vi "LDO Terminate Conditions.vi"(8 "error in (no error)":errorcluster, 10 "Event Booleans":T1, 11 "All Data":T2 {"PLC Data"."PLC Data - LDO"."Timing"."Absolute Time" format="%<%H:%M:%S%3u>t"; "PLC Data"."PLC Data - LDO"."Timing"."Display Time" format="%#.20f"; "PLC Data"."PLC Data - LDO"."Timing"."Test Time Ref" format="%#.20f"; "PLC Data"."PLC Data - LDO"."Timing"."Precondition Time Ref" format="%#.20f"; "PLC Data"."PLC Data - LDO"."Timing"."First Call Time Ref" format="%#.20f"; "PLC Data"."PLC Data - FVIR"."Timing"."Absolute Time" format="%<%H:%M:%S%3u>t"; "PLC Data"."PLC Data - FVIR"."Timing"."Display Time" format="%#.20f"; "PLC Data"."PLC Data - FVIR"."Timing"."Test Time Ref" format="%#.20f"; "PLC Data"."PLC Data - FVIR"."Timing"."Precondition Time Ref" format="%#.20f"; "PLC Data"."PLC Data - FVIR"."Timing"."First Call Time Ref" format="%#.20f"}) -> (0 "error out":errorcluster, 2 "Event Booleans Out":T1, 3 "All Data Out":T2 {"PLC Data"."PLC Data - LDO"."Timing"."Absolute Time" format="%<%H:%M:%S%3u>t"; "PLC Data"."PLC Data - LDO"."Timing"."Display Time" format="%#.20f"; "PLC Data"."PLC Data - LDO"."Timing"."Test Time Ref" format="%#.20f"; "PLC Data"."PLC Data - LDO"."Timing"."Precondition Time Ref" format="%#.20f"; "PLC Data"."PLC Data - LDO"."Timing"."First Call Time Ref" format="%#.20f"; "PLC Data"."PLC Data - FVIR"."Timing"."Absolute Time" format="%<%H:%M:%S%3u>t"; "PLC Data"."PLC Data - FVIR"."Timing"."Display Time" format="%#.20f"; "PLC Data"."PLC Data - FVIR"."Timing"."Test Time Ref" format="%#.20f"; "PLC Data"."PLC Data - FVIR"."Timing"."Precondition Time Ref" format="%#.20f"; "PLC Data"."PLC Data - FVIR"."Timing"."First Call Time Ref" format="%#.20f"})   [LabVIEW 2020]
uses:
  Modbus/Modbus All Data.ctl
  Modbus/Modbus PLC Data All.ctl
  Modbus/Modbus FVIR Control.ctl
  Modbus/Modbus Timing.ctl
  <vilib>/Utility/miscctls.llb/LVDateTimeRec.ctl
  Modbus/Modbus LDO Control.ctl
  WritingDataFile/Data to Save.ctl
  Terminate Conditions Cluster.ctl
  Drivers/Inficon Transmitter/Type Definitions/Inficon Data.ctl
  Modbus/Modbus Gas Meter Data.ctl
  Drivers/Alicat LabVIEW Drivers 2v1/Sub-VIs/Data Cluster.ctl
  Drivers/Alicat LabVIEW Drivers 2v1/Sub-VIs/Units of Measure.ctl
  Gas_Rate/HEWH ANSI Rate.ctl
  Drivers/Resideo Gas Valve/Type Definitions/Vesta Info.ctl
  Event Booleans.ctl
panel:
  # "Totalizer Timer"
  # "Totalizer Timer"
  # "Natural Gas"
  # "Propane"
  # "Totalizer Timer"
  # "Totalizer Timer"
  # "Natural Gas"
  # "Propane"
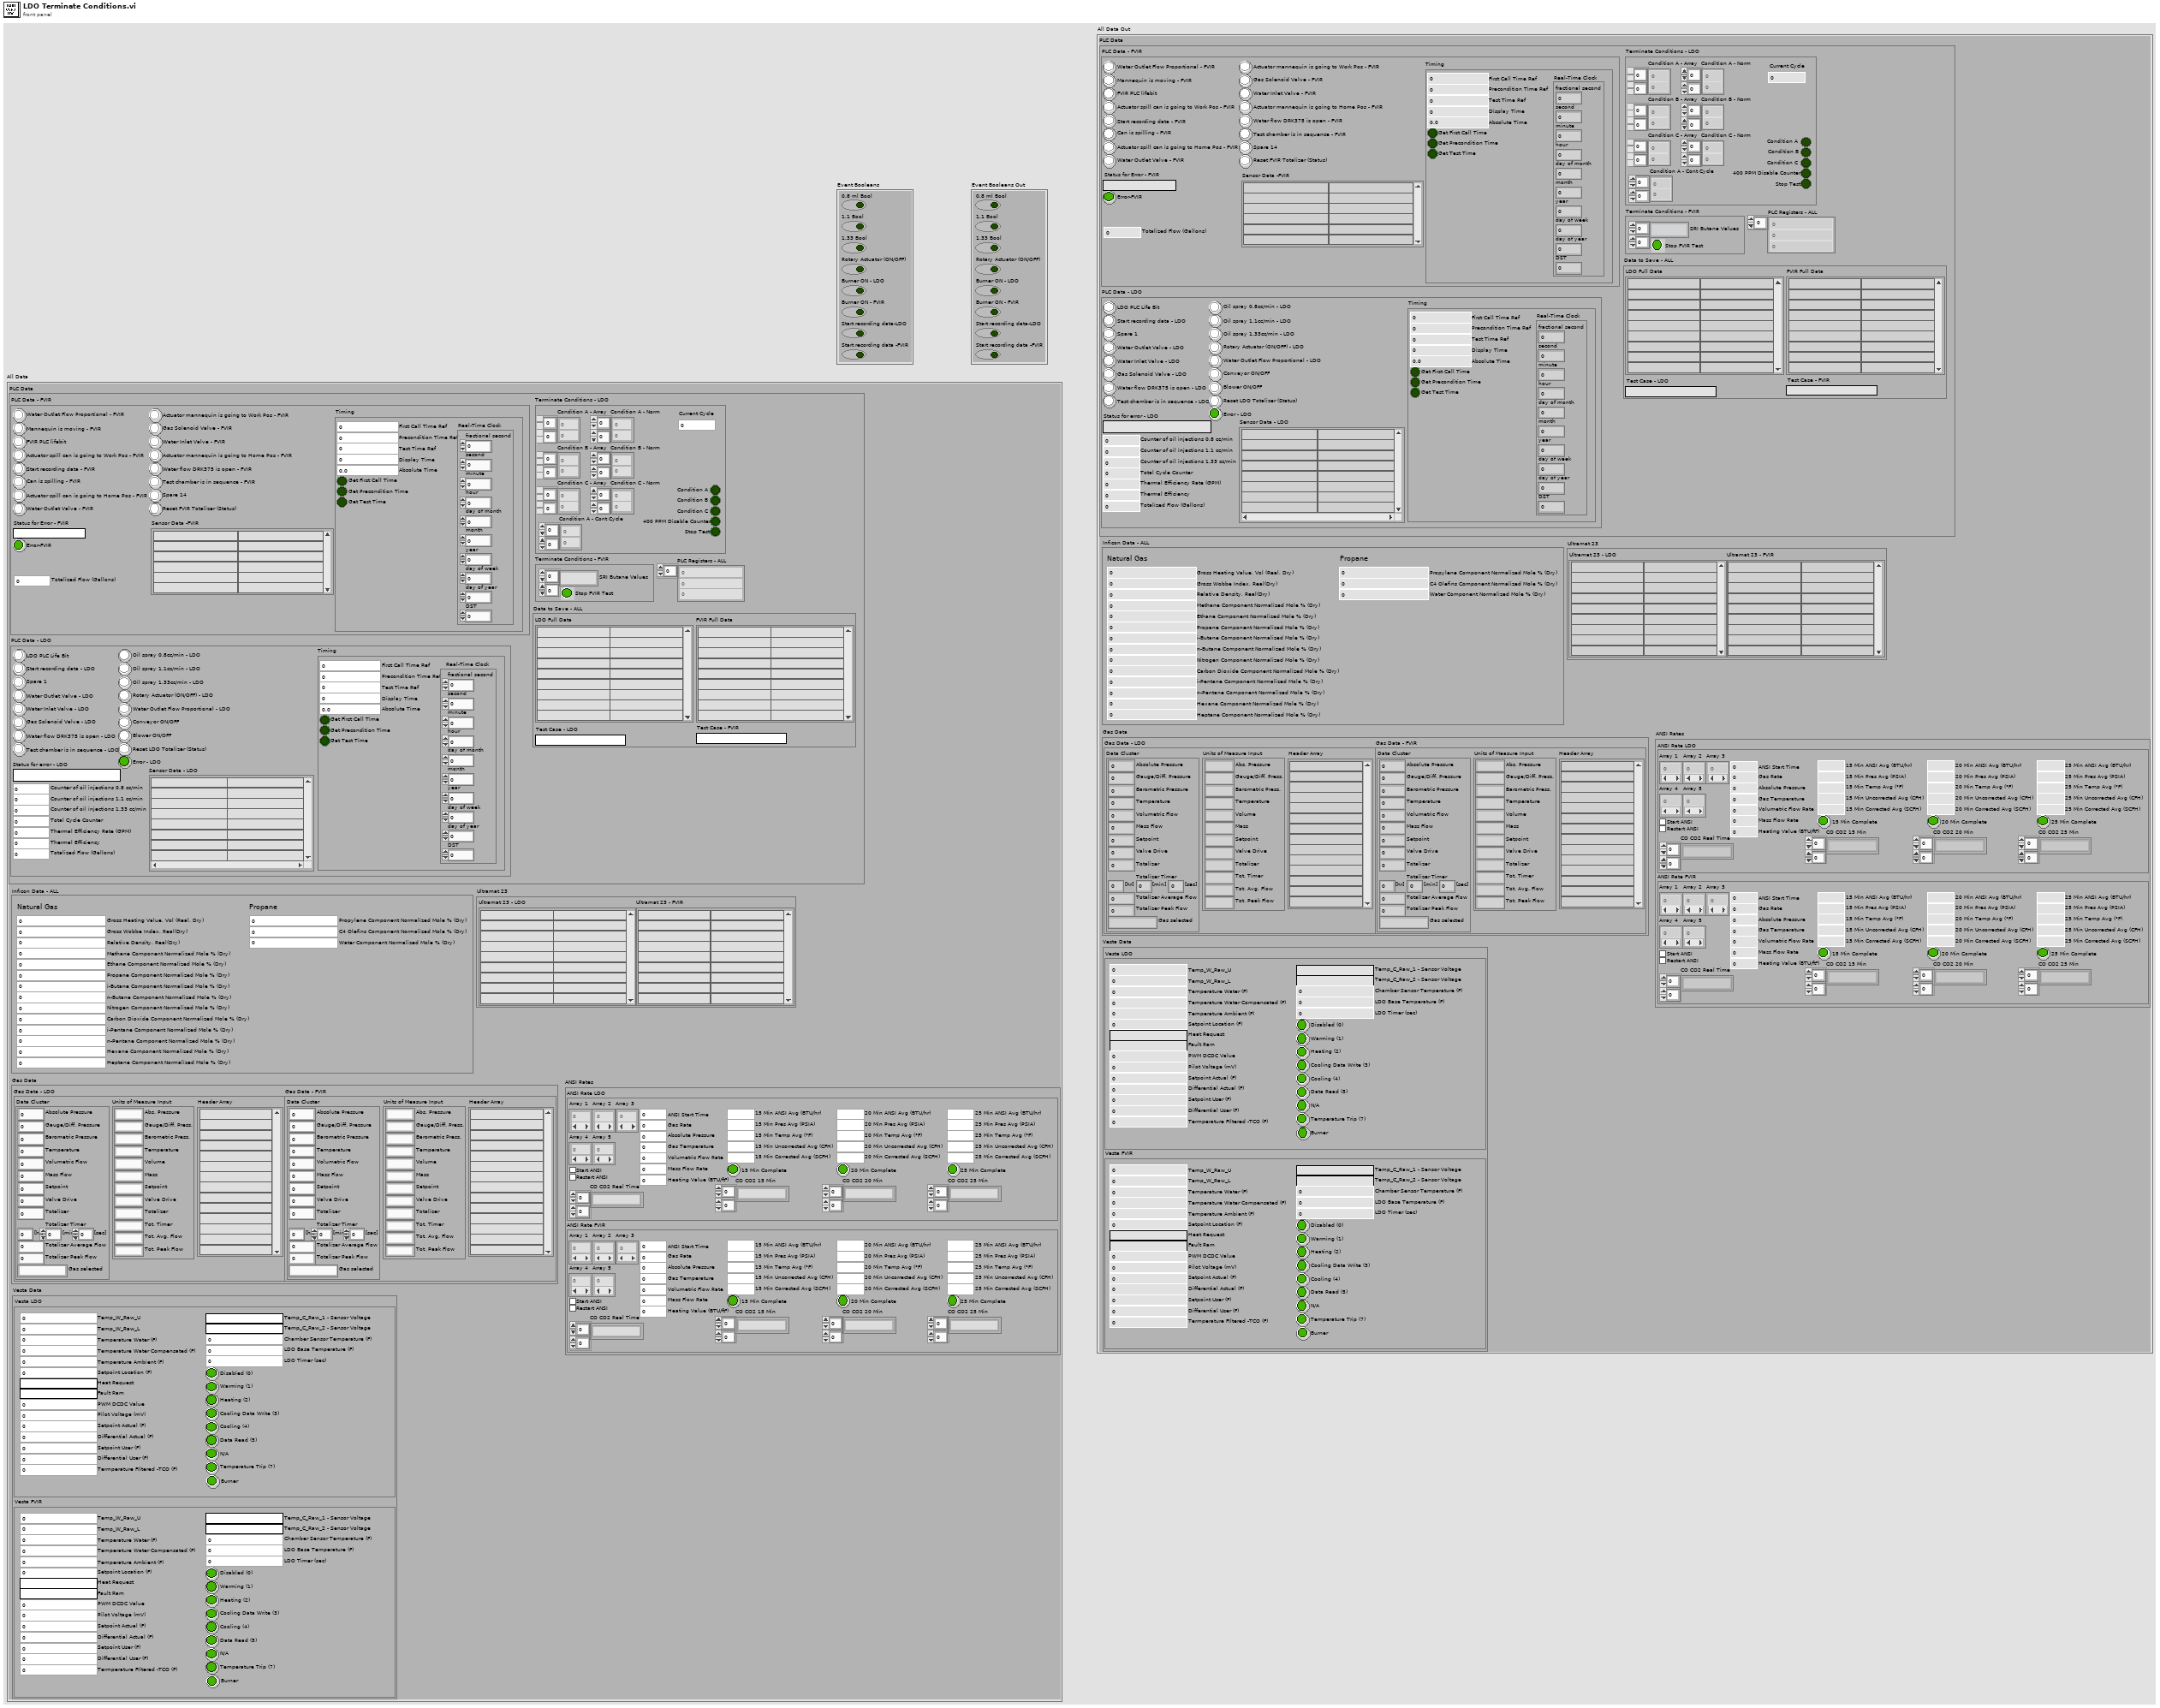
[diagram p1: front panel]
types:
  T1 = typedef "Event Booleans.ctl" = cluster{"Burner ON - LDO":bool, "0.8 ml Bool":bool, "1.1 Bool":bool, "1.33 Bool":bool, "Start recording data-LDO":bool, "Rotary Actuator (ON/OFF)":bool, "Burner ON - FVIR":bool, "Start recording data -FVIR ":bool}
  T2 = typedef "Modbus All Data.ctl" = cluster{"PLC Data":T3, "Inficon Data - ALL":T10, "Gas Data":cluster{"Gas Data - LDO":T11, "Gas Data - FVIR":T11}, "Ultramat 23":cluster{"Ultramat 23 - LDO":string[][], "Ultramat 23 - FVIR":string[][]}, "ANSI Rates":cluster{"ANSI Rate LDO":T14, "ANSI Rate FVIR":T14}, "Vesta Data":cluster{"Vesta LDO":T15, "Vesta FVIR":T15}}
  T3 = typedef "Modbus PLC Data All.ctl" = cluster{"PLC Data - FVIR":T4, "PLC Data - LDO":T7, "PLC Registers - ALL":i16[], "Data to Save - ALL":T8, "Terminate Conditions - LDO":T9, "Terminate Conditions - FVIR":cluster{"SRI Butane Values":string[][], "Stop FVIR Test":bool}}
  T4 = typedef "Modbus FVIR Control.ctl" = cluster{"Reset FVIR Totalizer (Status)":bool, "Spare 14":bool, "Actuator mannequin is going to Work Pos - FVIR":bool, "Actuator mannequin is going to Home Pos - FVIR":bool, "Test chamber is in sequence - FVIR ":bool, "Water flow DRK375 is open - FVIR":bool, "Gas Solenoid Valve - FVIR":bool, "Water Inlet Valve - FVIR":bool, "Water Outlet Flow Proportional - FVIR":bool, "Start recording data - FVIR":bool, "Actuator spill can is going to Work Pos - FVIR":bool, "Actuator spill can is going to Home Pos - FVIR":bool, "Water Outlet Valve - FVIR":bool, "Can is spilling - FVIR":bool, "Mannequin is moving - FVIR":bool, "FVIR PLC lifebit":bool, "Status for Error - FVIR":string, "Error-FVIR":bool, "Sensor Data -FVIR":string[][], "Totalized Flow (Gallons)":dbl, "Timing":T5}
  T5 = typedef "Modbus Timing.ctl" = cluster{"First Call Time Ref":dbl, "Precondition Time Ref":dbl, "Test Time Ref":dbl, "Get First Call Time":bool, "Get Precondition Time":bool, "Get Test Time":bool, "Display Time":dbl, "Real-Time Clock":T6, "Absolute Time":dbl}
  T6 = typedef "LVDateTimeRec.ctl" = cluster{"fractional second":dbl, "second":i32, "minute":i32, "hour":i32, "day of month":i32, "month":i32, "year":i32, "day of week":i32, "day of year":i32, "DST":i32}
  T7 = typedef "Modbus LDO Control.ctl" = cluster{"LDO PLC Life Bit":bool, "Start recording data - LDO":bool, "Spare 1":bool, "Water Outlet Valve - LDO":bool, "Water Inlet Valve - LDO":bool, "Gas Solenoid Valve - LDO":bool, "Water flow DRK375 is open - LDO":bool, "Test chamber is in sequence - LDO":bool, "Oil spray 0.8cc/min - LDO":bool, "Oil spray 1.1cc/min - LDO":bool, "Oil spray 1.33cc/min - LDO":bool, "Rotary Actuator (ON/OFF) - LDO":bool, "Water Outlet Flow Proportional - LDO":bool, "Conveyor ON/OFF":bool, "Blower ON/OFF":bool, "Reset LDO Totalizer (Status)":bool, "Status for error - LDO":string, "Error - LDO":bool, "Sensor Data - LDO":string[][], "Thermal Efficiency Rate (GPM)":dbl, "Thermal Efficiency":dbl, "Totalized Flow (Gallons)":dbl, "Counter of oil injections 1.33 cc/min":u16, "Total Cycle Counter":u16, "Counter of oil injections 1.1 cc/min":u16, "Counter of oil injections 0.8 cc/min":u16, "Timing":T5}
  T8 = typedef "Data to Save.ctl" = cluster{"LDO Full Data":string[][], "FVIR Full Data":string[][], "Test Case - FVIR":string, "Test Case - LDO":string}
  T9 = typedef "Terminate Conditions Cluster.ctl" = cluster{"Condition B - Array":dbl[][], "Current Cycle":u16, "Condition C - Array":dbl[][], "Condition A - Array":dbl[][], "400 PPM Disable Counter":bool, "Condition A - Norm":dbl[][], "Condition B - Norm":dbl[][], "Condition C - Norm":dbl[][], "Condition A":bool, "Condition B":bool, "Condition C":bool, "Condition A - Cont Cycle":dbl[][], "Stop Test":bool}
  T10 = typedef "Inficon Data.ctl" = cluster{"Gross Heating Value, Vol (Real, Dry)":dbl, "Nitrogen Component Normalized Mole % (Dry)":dbl, "Methane Component Normalized Mole % (Dry)":dbl, "Carbon Dioxide Component Normalized Mole % (Dry)":dbl, "Ethane Component Normalized Mole % (Dry)":dbl, "Propane Component Normalized Mole % (Dry)":dbl, "i-Pentane Component Normalized Mole % (Dry)":dbl, "i-Butane Component Normalized Mole % (Dry)":dbl, "n-Butane Component Normalized Mole % (Dry)":dbl, "n-Pentane Component Normalized Mole % (Dry)":dbl, "Hexane Component Normalized Mole % (Dry)":dbl, "Heptane Component Normalized Mole % (Dry)":dbl, "Gross Wobbe Index, Real(Dry)":dbl, "Relative Density, Real(Dry)":dbl, "Propylene Component Normalized Mole % (Dry)":dbl, "C4 Olefins Component Normalized Mole % (Dry)":dbl, "Water Component Normalized Mole % (Dry)":dbl}
  T11 = typedef "Modbus Gas Meter Data.ctl" = cluster{"Data Cluster":T12, "Units of Measure Input":T13, "Header Array":string[]}
  T12 = typedef "Data Cluster.ctl" = cluster{"Absolute Pressure":dbl, "Gauge/Diff. Pressure":dbl, "Barometric Pressure":dbl, "Temperature":dbl, "Volumetric Flow":dbl, "Mass Flow":dbl, "Setpoint":dbl, "Valve Drive":dbl, "Totalizer":dbl, "[hr]":dbl, "[min]":dbl, "[sec]":dbl, "Totalizer Average Flow":dbl, "Totalizer Peak Flow":dbl, "Gas selected":string}
  T13 = typedef "Units of Measure.ctl" = cluster{"Abs. Pressure":string, "Gauge/Diff. Press.":string, "Barometric Press.":string, "Temperature":string, "Volume":string, "Mass":string, "Setpoint":string, "Valve Drive":string, "Totalizer":string, "Tot. Timer":string, "Tot. Avg. Flow":string, "Tot. Peak Flow":string}
  T14 = typedef "HEWH ANSI Rate.ctl" = cluster{"Array 1":dbl[], "Array 3":dbl[], "Array 2":dbl[], "Start ANSI":bool, "ANSI Start Time":dbl, "Restart ANSI":bool, "15 Min ANSI Avg (BTU/hr)":dbl, "20 Min ANSI Avg (BTU/hr)":dbl, "25 Min ANSI Avg (BTU/hr)":dbl, "Absolute Pressure":dbl, "Gas Temperature":dbl, "Volumetric Flow Rate":dbl, "Mass Flow Rate":dbl, "Array 4":dbl[], "Array 5":dbl[], "Gas Rate":dbl, "15 Min Pres Avg (PSIA)":dbl, "20 Min Pres Avg (PSIA)":dbl, "25 Min Pres Avg (PSIA)":dbl, "15 Min Temp Avg (°F) ":dbl, "20 Min Temp Avg (°F)":dbl, "25 Min Temp Avg (°F)":dbl, "15 Min Uncorrected Avg (CFH)":dbl, "20 Min Uncorrected Avg (CFH)":dbl, "25 Min Uncorrected Avg (CFH)":dbl, "15 Min Corrected Avg (SCFH)":dbl, "20 Min Corrected Avg (SCFH)":dbl, "25 Min Corrected Avg (SCFH)":dbl, "15 Min Complete":bool, "20 Min Complete":bool, "25 Min Complete":bool, "Heating Value (BTU/ft³)":dbl, "CO CO2 15 Min":string[][], "CO CO2 20 Min":string[][], "CO CO2 25 Min":string[][], "CO CO2 Real Time":string[][]}
  T15 = typedef "Vesta Info.ctl" = cluster{"Temp_W_Raw_U":u16, "Temp_W_Raw_L":u16, "Temperature Water (F)":dbl, "Temperature Water Compensated (F)":dbl, "Temperature Ambient (F)":dbl, "Setpoint Location (F)":dbl, "Heat Request":string, "Fault Ram":string, "PWM DCDC Value":u16, "Pilot Voltage (mV)":dbl, "Setpoint Actual (F)":dbl, "Differential Actual (F)":dbl, "Setpoint User (F)":dbl, "Differential User (F)":dbl, "Termperature FIltered -TCO (F)":dbl, "Temp_C_Raw_1 - Sensor Voltage":string, "Temp_C_Raw_2 - Sensor Voltage":string, "Chamber Sensor Temperature (F)":dbl, "LDO Base Temperature (F)":dbl, "LDO Timer (sec)":i16, "Disabled (0)":bool, "Warming (1)":bool, "Heating (2)":bool, "Cooling Data Write (3)":bool, "Cooling (4)":bool, "Data Read (5)":bool, "N/A":bool, "Temperature Trip (7)":bool, "Burner":bool}
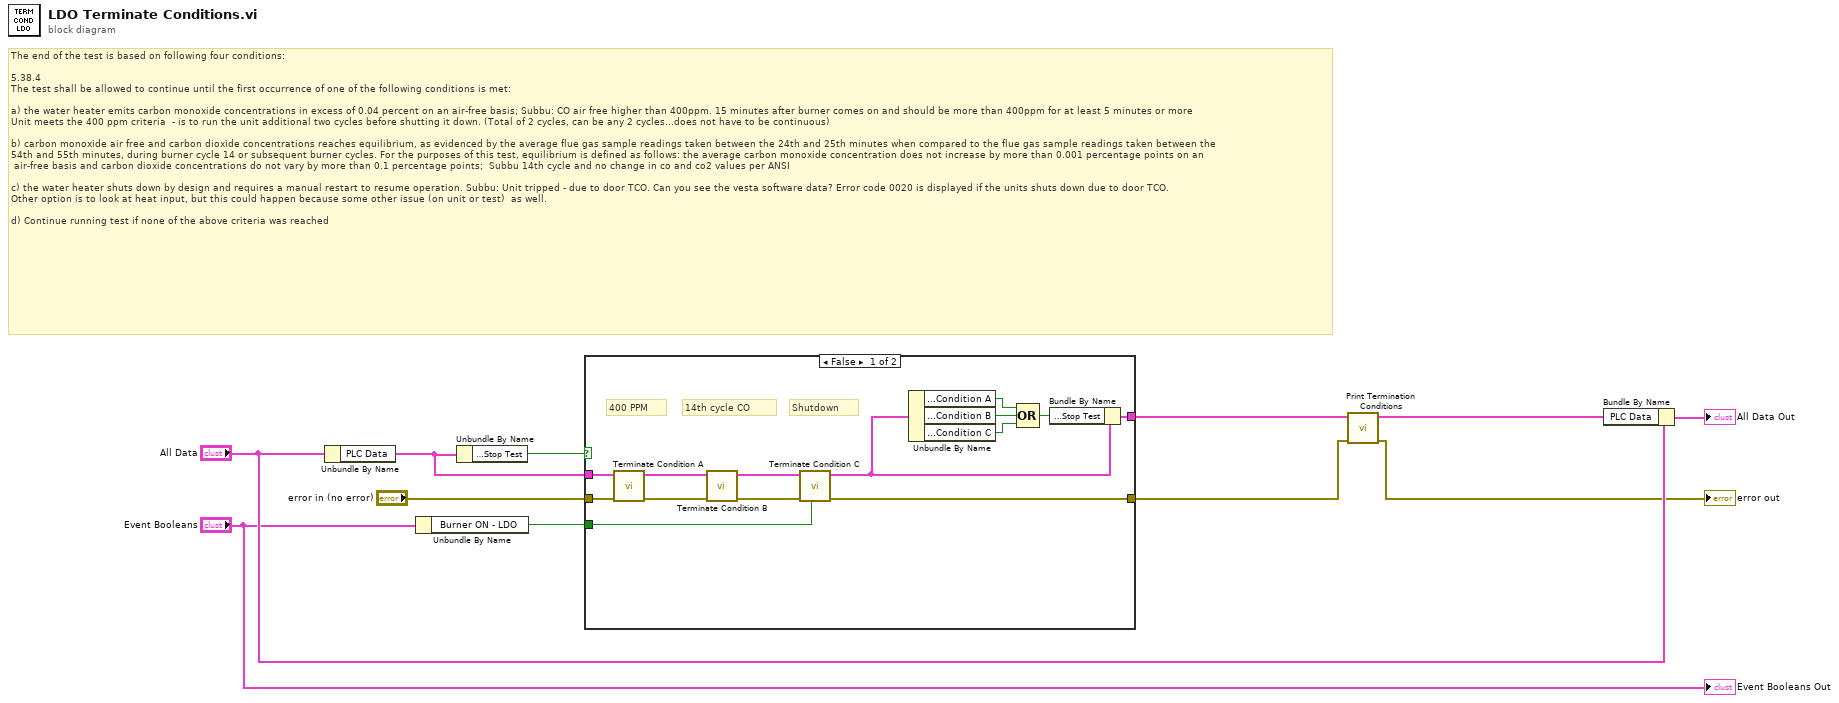
[diagram p0: block diagram]
diagram:
  # "The end of the test is based on following four conditions:\n\n5.38.4\nThe test shall be allowed to continue until the first occurrence of one of the following conditions is met: \n\na) the water heater emits carbon monoxide concentrations in excess of 0.04 percent on an air-free basis; Subbu: CO air free higher than 400ppm. 15 minutes after burner comes on and should be more than 400ppm for at least 5 minutes or more\nUnit meets the 400 ppm criteria  - is to run the unit additional two cycles before shutting it down. (Total of 2 cycles, can be any 2 cycles...does not have to be continuous)\n\nb) carbon monoxide air free and carbon dioxide concentrations reaches equilibrium, as evidenced by the average flue gas sample readings taken between the 24th and 25th minutes when compared to the flue gas sample readings taken between the\n54th and 55th minutes, during burner cycle 14 or subsequent burner cycles. For the purposes of this test, equilibrium is defined as follows: the average carbon monoxide concentration does not increase by more than 0.001 percentage points on an\n air-free basis and carbon dioxide concentrations do not vary by more than 0.1 percentage points;  Subbu 14th cycle and no change in co and co2 values per ANSI\n\nc) the water heater shuts down by design and requires a manual restart to resume operation. Subbu: Unit tripped - due to door TCO. Can you see the vesta software data? Error code 0020 is displayed if the units shuts down due to door TCO. \nOther option is to look at heat input, but this could happen because some other issue (on unit or test)  as well.\n\nd) Continue running test if none of the above criteria was reached"
  n1 = Unbundle By Name("All Data") -> ("PLC Data"=w9:T3)
  n2 = Unbundle By Name("Event Booleans") -> ("Burner ON - LDO"=w6:bool)
  n3 = Unbundle By Name(w9) -> ("Terminate Conditions - LDO.Stop Test"=w10:bool)
  n4 = case shown="False" w10 {
    tunnel: w6 -> [w25 _]
    tunnel: w9 -> [w24 w27]
    tunnel: [w21 w26] -> w2
    tunnel: "error in (no error)" -> [w20 w26]
    tunnel: [w13 w27] -> w4
    frame False {
      # "Shutdown"
      # "14th cycle CO"
      # "400 PPM"
      n5 = call "Terminate Condition A.vi"("error in"=w20, "PLC Data In"=w24) -> ("error out"=w23:errorcluster, "PLC Data Out"=w19:T3)  [unwired: 8 in]
      n6 = call "Terminate Condition B.vi"("error in (no error)"=w23, "PLC Data Out in"=w19) -> ("error out"=w22:errorcluster, "PLC Data Out out"=w18:T3)  [unwired: 8 in]
      n7 = call "Terminate Condition C.vi"("Burner ON"=w25, "error in"=w22, "PLC Data In"=w18) -> ("error out"=w21:errorcluster, "PLC Data Out"=w14:T3)  [unwired: 7 in]
      n8 = Unbundle By Name(w14) -> ("Terminate Conditions - LDO.Condition A"=w17:bool, "Terminate Conditions - LDO.Condition B"=w16:bool, "Terminate Conditions - LDO.Condition C"=w15:bool)
      n9 = Compound Arithmetic op=OR(w17, w16, w15) -> (w12:bool)
      n10 = Bundle By Name(cluster=w14, "Terminate Conditions - LDO.Stop Test"=w12) -> (w13:T3)
    }
    frame True {
    }
  }
  n11 = call "Print Termination Conditions.vi"("error in"=w2, "PLC Data"=w4) -> ("error out"=→"error out":errorcluster, "PLC Data Output"=w3:T3)  [unwired: 8 in]
  n12 = Bundle By Name(cluster="All Data", "PLC Data"=w3) -> (→"All Data Out":T2)
  "Event Booleans Out" <- "Event Booleans"
